vi "Save_teplete(Subvi).vi"(9 "숫자형":i32, 11 "배열":string[](array[string])) -> ()   [LabVIEW 2024]
uses:
  <vilib>/Utility/sysdir.llb/System Directory Type.ctl
  <vilib>/Utility/file.llb/Write Delimited Spreadsheet (string).vi
panel:
  out "참조 번호 출력 4":refnum<file>
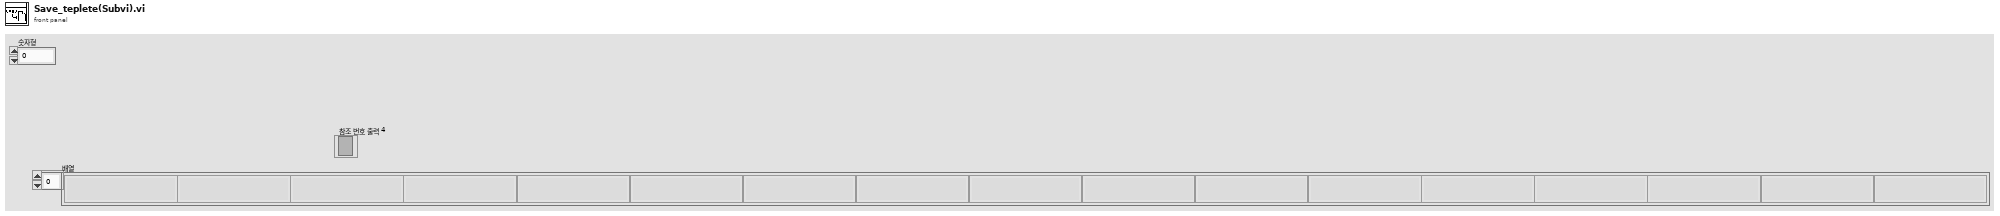
[diagram p1: front panel]
types:
  T1 = enum16{"open", "replace", "create", "open or create", "replace or create", "replace or create with confirmation"}
  T2 = typedef "System Directory Type.ctl" = i32
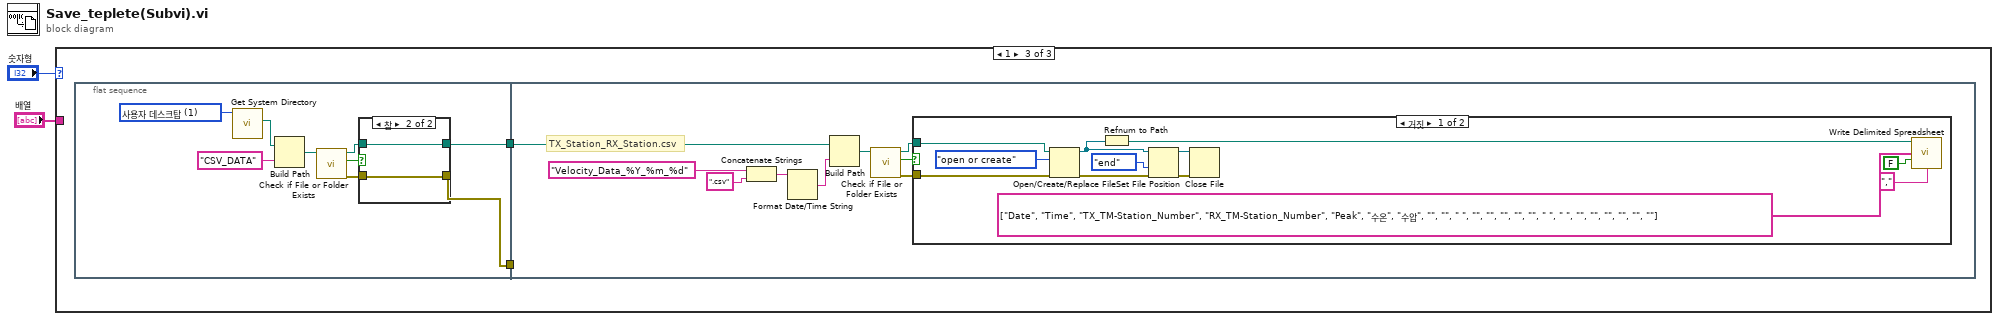
[diagram p0: block diagram]
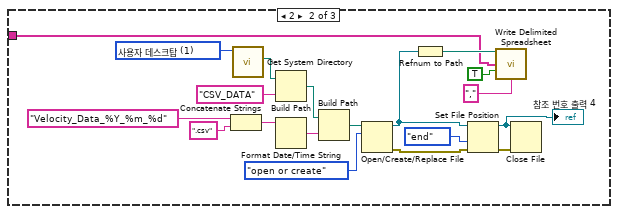
[diagram p3: hidden frame]
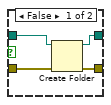
[diagram p4: hidden frame]
diagram:
  n1 = case shown="1" "숫자형" {
    tunnel: "배열" -> [_ w3 _]
    frame Default {
    }
    frame 2 {
      w19 = T2 1 items=["사용자 홈"=0, "사용자 데스크탑"=1, "사용자 문서"=2, "사용자 어플리케이션 데이터"=3, "사용자 환경"=4, "사용자 임시"=5, "퍼블릭 문서"=6, "퍼블릭 어플리케이션 데이터"=7, "퍼블릭 환경"=8, "퍼블릭 캐시"=13, "시스템 코어 라이브러리"=9, "시스템 설치된 라이브러리"=10, "어플리케이션 파일"=11, "부팅 볼륨 루트"=12] ("system directory type")
      n2 = Concatenate Strings("Velocity_Data_%Y_%m_%d" ("시간 포맷 문자열 (%c)"), ".csv" ("시간 포맷 문자열 (%c)")) -> (w6:string)
      n3 = call <vilib>:"Get System Directory.vi"("system directory type"=w19) -> ("system directory"=w4:path)  [unwired: 10 in]
      n4 = Build Path(base path=w4, name or relative path="CSV_DATA") -> (appended path=w20:path)
      n5 = Format Date/Time String(time format string (%c)=w6) -> (date/time string=w5:string)  [unwired: 2 in]
      n6 = Build Path(base path=w20, name or relative path=w5) -> (appended path=w21:path)
      n7 = Open/Create/Replace File(file path (use dialog)=w21, operation (0:open)=T1."open or create" ("동작(0:open)")) -> (refnum out=w10:refnum<file>, error out=w8:errorcluster)  [unwired: 4 in, 1 out]
      n8 = Refnum to Path(1:w10) -> (0:w11:path)
      n9 = Set File Position(refnum=w10, from (0:start)=enum16{"start", "end", "current"}."end" ("위치(0:start)"), error in=w8) -> (refnum out=w9:refnum<file>, error out=w7:errorcluster)  [unwired: 1 in]
      "참조 번호 출력 4" <- w9
      n10 = call-poly <vilib>:"Write Delimited Spreadsheet.vi"("file path (dialog if empty)"=w11, "1D data"=w3, "append to file? (new file:F)"=TRUE, "delimiter (\\t)"="," ("delimiter (\\t)")) -> ()  [unwired: 10 in, 2 out]
      n11 = Close File(refnum=w9, error in=w7) -> ()  [unwired: 2 out]
    }
    frame 1 {
      n12 = flat-sequence {
        tunnel: [w25] -> w23
        tunnel: [w24] -> w22
        tunnel: w23 -> [w43]
        tunnel: w22 -> [_]
        frame #0 {
          w32 = T2 1 items=["사용자 홈"=0, "사용자 데스크탑"=1, "사용자 문서"=2, "사용자 어플리케이션 데이터"=3, "사용자 환경"=4, "사용자 임시"=5, "퍼블릭 문서"=6, "퍼블릭 어플리케이션 데이터"=7, "퍼블릭 환경"=8, "퍼블릭 캐시"=13, "시스템 코어 라이브러리"=9, "시스템 설치된 라이브러리"=10, "어플리케이션 파일"=11, "부팅 볼륨 루트"=12] ("system directory type")
          n13 = call <vilib>:"Get System Directory.vi"("system directory type"=w32) -> ("system directory"=w26:path)  [unwired: 10 in]
          n14 = Build Path(base path=w26, name or relative path="CSV_DATA") -> (appended path=w30:path)
          n15 = call <vilib>:"Check if File or Folder Exists.vi"("path"=w30) -> ("error out"=w29:errorcluster, "file or folder exists?"=w27:bool, "dup path"=w28:path)  [unwired: 8 in]
          n16 = case shown="참" w27 {
            tunnel: w28 -> [w36 w38]
            tunnel: w29 -> [w35 w37]
            tunnel: [w34 w38] -> w25
            tunnel: [w33 w37] -> w24
            frame False {
              n17 = Create Folder(path (use dialog)=w36, error in=w35) -> (created path=w34:path, error out=w33:errorcluster)  [unwired: 1 in, 1 out]
            }
            frame True {
            }
          }
        }
        frame #1 {
          # "TX_Station_RX_Station.csv"
          n18 = Concatenate Strings("Velocity_Data_%Y_%m_%d" ("시간 포맷 문자열 (%c)"), ".csv" ("시간 포맷 문자열 (%c)")) -> (w46:string)
          n19 = Format Date/Time String(time format string (%c)=w46) -> (date/time string=w44:string)  [unwired: 2 in]
          n20 = Build Path(base path=w43, name or relative path=w44) -> (appended path=w42:path)
          n21 = call <vilib>:"Check if File or Folder Exists.vi"("path"=w42) -> ("error out"=w39:errorcluster, "file or folder exists?"=w41:bool, "dup path"=w40:path)  [unwired: 8 in]
          n22 = case shown="거짓" w41 {
            tunnel: w40 -> [w54 _]
            tunnel: w39 -> [w53 _]
            frame False {
              n23 = Open/Create/Replace File(file path (use dialog)=w54, error in=w53, operation (0:open)=T1."open or create" ("동작(0:open)")) -> (refnum out=w48:refnum<file>, error out=w58:errorcluster)  [unwired: 3 in, 1 out]
              n24 = Refnum to Path(1:w48) -> (0:w52:path)
              n25 = Set File Position(refnum=w48, from (0:start)=enum16{"start", "end", "current"}."end" ("위치(0:start)"), error in=w58) -> (refnum out=w59:refnum<file>, error out=w57:errorcluster)  [unwired: 1 in]
              n26 = Close File(refnum=w59, error in=w57) -> ()  [unwired: 2 out]
              n27 = call-poly <vilib>:"Write Delimited Spreadsheet.vi"("file path (dialog if empty)"=w52, "1D data"=string[] ["Date", "Time", "TX_TM-Station_Number", "RX_TM-Station_Number", "Peak", "수온", "수압", "", "", " ", "", "", "", "", "", " ", " ", "", "", "", "", "", ""], "append to file? (new file:F)"=FALSE, "delimiter (\\t)"="," ("delimiter (\\t)")) -> ()  [unwired: 10 in, 2 out]
            }
            frame True {
            }
          }
        }
      }
    }
  }
